vi "LINC Register Callback.vi"(8 "error in (no error)":errorcluster, 9 "callback ref":refnum<vi>, 10 "mode (cmd)":enum16{"CMD", "TLM"}(ring), 11 "LINC session":refnum<class "LINC.lvclass">) -> (0 "error out":errorcluster, 3 "dup LINC session":refnum<class "LINC.lvclass">)   [LabVIEW 2018, in "STEPkgDriver_LINC.lvlib" / "LINC.lvclass"]
uses:
  LINC.lvclass
  STEPkgDriver_LINC.lvlib
  LINC Config.ctl
  LINC Global Config Mode.ctl
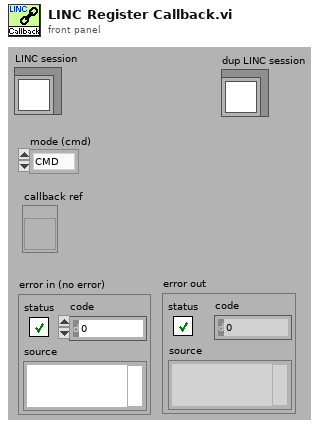
[diagram p1: front panel]
types:
  T1 = typedef "STEPkgDriver_LINC.lvlib/LINC Global Config Mode.ctl" = enum16{"INIT", "CLEAR", "SET_CMD_CB", "SET_TLM_CB", "SET_CMD_FIELDS", "SET_TLM_FIELDS", "SET_ID", "GET_CONFIG"}
  T2 = typedef "STEPkgDriver_LINC.lvlib/LINC Config.ctl" = cluster{"cmd callback":refnum<vi>, "tlm callback":refnum<vi>, "cmd ID bitoffset":i32, "cmd ID bitsize":i32, "cmd IDs":i32[], "tlm ID bitoffset":i32, "tlm ID bitsize":i32, "tlm IDs":i32[], "cmd header fields":i32, "tlm header fields":i32, "tlm header size":i32}
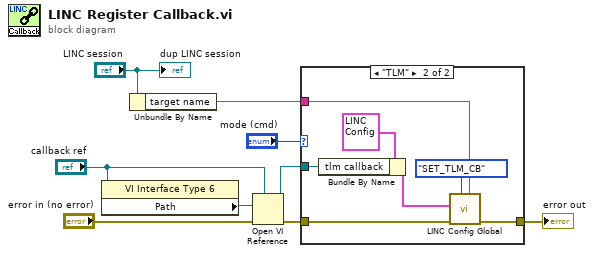
[diagram p0: block diagram]
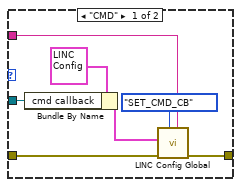
[diagram p2: hidden frame]
diagram:
  n1 = property class="VI Interface Type 6"(reference="callback ref") -> ("Path"=w8:path)  [unwired: 1 in, 2 out]
  n2 = Unbundle By Name("LINC session") -> ("target name"=w4:string)
  n3 = Open VI Reference(type specifier VI Refnum (for type only)="callback ref", vi path=w8, error in (no error)="error in (no error)") -> (vi reference=w3:refnum<vi>, error out=w6:errorcluster)  [unwired: 3 in]
  n4 = case shown="\"TLM\"" "mode (cmd)" {
    tunnel: w6 -> [w16 w23]
    tunnel: [w15 w22] -> w5
    tunnel: w4 -> [w14 w21]
    tunnel: w3 -> [w11 w18]
    frame "CMD" {
      n5 = Bundle By Name(cluster=T2 {"cmd callback"=refnum, "tlm callback"=refnum, "cmd ID bitoffset"=0, "cmd ID bitsize"=0, "cmd IDs"=[], "tlm ID bitoffset"=0, "tlm ID bitsize"=0, "tlm IDs"=[], "cmd header fields"=0, "tlm header fields"=0, "tlm header size"=0} ("config in"), "cmd callback"=w11) -> (w12:T2)
      n6 = call "LINC Config Global.vi"("target name"=w14, "mode"=LINC_Global_Config_Mode."SET_CMD_CB", "error in (no error)"=w16, "config in"=w12) -> ("error out"=w15:errorcluster)  [unwired: 6 in, 1 out]
    }
    frame "TLM" {
      n7 = Bundle By Name(cluster=T2 {"cmd callback"=refnum, "tlm callback"=refnum, "cmd ID bitoffset"=0, "cmd ID bitsize"=0, "cmd IDs"=[], "tlm ID bitoffset"=0, "tlm ID bitsize"=0, "tlm IDs"=[], "cmd header fields"=0, "tlm header fields"=0, "tlm header size"=0} ("config in"), "tlm callback"=w18) -> (w19:T2)
      n8 = call "LINC Config Global.vi"("target name"=w21, "mode"=LINC_Global_Config_Mode."SET_TLM_CB", "error in (no error)"=w23, "config in"=w19) -> ("error out"=w22:errorcluster)  [unwired: 6 in, 1 out]
    }
  }
  "error out" <- w5
  "dup LINC session" <- "LINC session"
